vi "Dashboard Main.vi"() -> ()   [LabVIEW 2019]
uses:
  <vilib>/Utility/miscctls.llb/LVRowAndColumnTypeDef.ctl
  <vilib>/event_ctls.llb/eventvkey.ctl
  <vilib>/Rock Robotics/Network Tables/NT Read Numeric Array.vi
  <vilib>/Rock Robotics/WPI/Dashboard/WPI_DashboardLogging Global.vi
  <vilib>/Rock Robotics/Network Tables/NT Read Boolean.vi
panel:
  out "Conveyor Sensor 3":bool
  out "Conveyor Sensor 2":bool
  out "Conveyor Sensor 4":bool
  out "Conveyor Sensor 1":bool
  in  "Camera Settings Right":T1={"Frame Rate"=30, "Compression"=30, "Size"=1, "DB Camera Config"=FALSE} {"Frame Rate" scale=1.0..30.0; "Compression" scale=100.0..-1.0; "Size" items=["640x480", "320x240", "160x120"]}
  in  "Camera Name Right":string(combo)="No Camera Selection"
  out "Camera Perf":string
  in  "Camera Settings":T1={"Frame Rate"=30, "Compression"=30, "Size"=1, "DB Camera Config"=FALSE} {"Frame Rate" scale=1.0..30.0; "Compression" scale=100.0..-1.0; "Size" items=["640x480", "320x240", "160x120"]}
  in  "TCP":refnum<k5>
  in  "Rec Mode":enum32{"Stop", "Record", "Playback"}(radio)
  out "Robot IP":string
  out "Image Message":string="Timeout in Camera Communications"
  in  "Dashboard Tab":T2(tab)
  in  "Select Auto":string(combo)="Select Autonomous ..."
  out "NT Connection":bool
  out "MotorChart R":cluster{"Numeric":dbl, "Numeric":dbl}(graph)
  out "MotorChart L":cluster{"Numeric":dbl, "Numeric":dbl}(graph)
  out "MotorSliders R":cluster{"MotorSlide1":dbl, "MotorSlide2":dbl} {"MotorSlide2" scale=-1.0..1.0 scale format="%#_2e"; "MotorSlide1" scale=-1.0..1.0 scale format="%#_2e"}
  out "MotorSliders L":cluster{"MotorSlide1":dbl, "MotorSlide2":dbl} {"MotorSlide2" scale=-1.0..1.0 scale format="%#_2e"; "MotorSlide1" scale=-1.0..1.0 scale format="%#_2e"}
  out "JS1 Z":dbl(slide) scale=-1.0..1.0 scale format="%#_2e"
  out "JS1 Graph":cluster{"X":dbl, "Y":dbl}[](graph)
  out "JS1 Buttons":T3
  out "JS2 Z":dbl(slide) scale=-1.0..1.0 scale format="%#_2e"
  out "JS2 Graph":cluster{"X":dbl, "Y":dbl}[](graph)
  out "JS2 Buttons":T3
  out "Mode":T4(ring)=enum."Auto Disabled"
  out "Right Camera Perf":cluster{"Bandwidth (Mbps)":dbl, "FPS":dbl}
  out "Camera Image Right":T5(plugin-control)
  in  "DB/String 9":string
  in  "DB/String 8":string
  in  "DB/String 7":string
  in  "DB/String 6":string
  in  "DB/String 5":string
  in  "DB/String 4":string
  in  "DB/String 3":string
  in  "DB/String 2":string
  in  "DB/String 1":string
  in  "DB/String 0":string
  in  "DB/Slider 0":dbl(slide) scale=0.0..5.0
  in  "DB/Slider 1":dbl(slide) scale=0.0..5.0
  in  "DB/Slider 2":dbl(slide) scale=0.0..5.0
  in  "DB/Slider 3":dbl(slide) scale=0.0..5.0
  out "DB/LED 3":bool
  out "DB/LED 2":bool
  out "DB/LED 1":bool
  out "DB/LED 0":bool
  in  "DB/Button 3":bool
  in  "DB/Button 2":bool
  in  "DB/Button 1":bool
  in  "DB/Button 0":bool caption="New Name"
  in  "Right MP Path":path
  in  "Left MP Path":path
  in  "Test Slider":dbl(slide) scale=0.0..100.0 scale format="%#_3g"
  in  "On/Off":bool caption="Solenoid"
  in  "Test Name":u16(ring) items=["Select the test to run..."]
  in  "Test Tree":string(tree)
  in  "Motor":cluster{"Value":dbl, "Enable":bool} {"Value" scale=-1.0..1.0 scale format="%#_3g"}
  out "Progress":T6 {"Test Progress" scale=0.0..100.0}
  in  "Rev/Fwd":cluster{"Forward":bool, "Reverse":bool}
  in  "Test Ring":u16(ring) items=["Monochrome", "Color"]
  out "Cmd Status":string
  in  "Execute Command":bool
  in  "Command Params":string[][](table)
  in  "Command Selection":i32(listbox)
  in  "CheckList":i32(listbox)
  out "Tree":string(tree)
  out "Camera Image":T5(plugin-control)
  in  "Camera Name":string(combo)="No Camera Selection"
  # "HW"
  # "HW"
  # "Joysticks"
  # "Drive Motors"
  # "Front"
  # "Right"
  # "Left"
  # "Back"
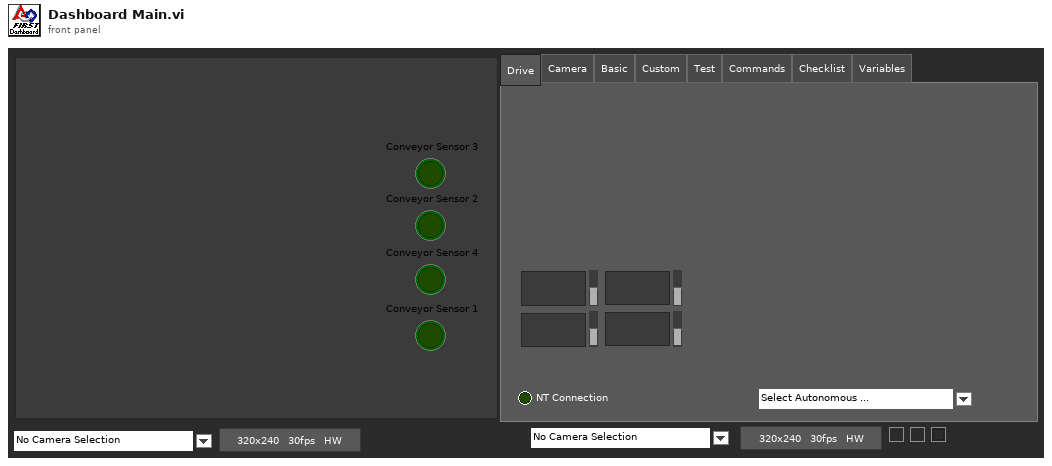
[diagram p1: front panel]
types:
  T1 = cluster{"Frame Rate":i32, "Compression":i32, "Size":u16, "DB Camera Config":bool}
  T2 = enum32{"Drive", "Camera", "Basic", "Custom", "Test", "Commands", "Checklist", "Variables"}
  T3 = cluster{bool, bool, bool, bool, bool, bool, bool, bool, bool, bool, bool, bool}
  T4 = enum8{"Tele-Op Disabled", "Tele-Op Enabled", "Auto Disabled", "Auto Enabled", "Test Disabled", "Test Enabled", "Disconnected", "No Code", "E-Stop"}
  T5 = typedef "IMAQ Image.ctl" = refnum<image>
  T6 = cluster{"Test Progress":u8, "Test Progress Text":string}
  T7 = enum16{"open", "replace", "create", "open or create", "replace or create", "replace or create with confirmation"}
  T8 = cluster{"Save Path":path, "Interval (s)":dbl, "Keep":i32}
  T9 = typedef "Image Type" = u32
  T10 = cluster{"IDs":cluster{"RPC field ID":u16, "Unique ID":u16}, "String":string}
  T11 = cluster{"Error Strings":string, "Disable Counts":cluster{u16, u16}, "Rail Faults":cluster{u16, u16, u16}, "Robot IP":string, "DB Mode":u8, "Event Info":cluster{"Name":string, "Type":u8, "Number":u16, "Replay":u8}}
  T12 = cluster{"Storage":cluster{"Disk Free":u64, "RAM Block":u32, "RAM free":u32}, "CPU Utilization":cluster{"CPU % ISR":sgl, "CPU % Time Crit":sgl, "CPU % Timed Str":sgl, "CPU % High":sgl, "CPU % Above":sgl, "CPU % Normal":sgl, "CPU % Low":sgl}, "CAN":cluster{"% Bus Utilization":sgl, "Bus Off Cnt":u32, "TX_FIFO Full Cnt":u32, "Receive Error Cnt":u8, "Transmit Error Cnt":u8}, "HID":cluster{"HID Outputs":u32, "Rumble Low":u16, "Rumble High":u16}[]}
  T13 = cluster{"Status bits":cluster{"Test Mode":bool, "Autonomous":bool, "Enabled":bool, "Code Start":bool, "Brownout":bool, "Reserved 2":bool, "Reserved 3":bool, "E-Stop":bool}, "Code Trace":cluster{"Disabled":bool, "TeleOp":bool, "Auto":bool, "Test":bool}, "Controller Type":enum16{"unknown", "cRIO", "roboRio"}, "Code?":enum16{"unknown", "noCode", "code"}, "Battery V":dbl}
  T14 = cluster{"Control Bits":cluster{"TestMode":bool, "Autonomous":bool, "Enabled":bool, "FMS Present":bool, bool, bool, bool, "E-Stop":bool}, "Team Station ":u8, "Countdown":sgl, "Joystick Values":cluster{"Axes":dbl[], "Buttons":bool[], "POVs":i16[]}[]}
  T15 = cluster{"Axes":dbl[], "Buttons":bool[], "POVs":i16[]}[]
  T16 = cluster{"Axes":dbl[], "Buttons":bool[], "POVs":i16[]}
  T17 = cluster{"Buttons[0]":bool, "Buttons[1]":bool, "Buttons[2]":bool, "Buttons[3]":bool, "Buttons[4]":bool, "Buttons[5]":bool, "Buttons[6]":bool, "Buttons[7]":bool, "Buttons[8]":bool, "Buttons[9]":bool, "Buttons[10]":bool, "Buttons[11]":bool}
  T18 = cluster{"Global Rectangle":i32[], "Contours":cluster{"Contour Type":u32, "ROI Type":u32, "Points":i32[]}[]}
  T19 = cluster{"Camera Name":string, string, "Saved DB Images Info":cluster{"Save Path":path, "Interval (s)":dbl, "Keep":i32}}
  T20 = cluster{"Camera Name Right":string, string, "Saved DB Images Info":cluster{"Save Path":path, "Interval (s)":dbl, "Keep":i32}}
  T21 = cluster{"Operation":enum16{"Update", "Clear"}, "Color Box":u32}[]
  T22 = typedef "eventvkey.ctl" = enum16{"ASCII", "Enter", "Return", "Shift", "Ctrl", "Alt", "Cmd", "Opt", "Caps", "NumLock", "Clear", "Break", "Up", "Down", "Left", "Right", "Insert", "Delete", "Home", "End", "PageUp", "PageDown", "Escape", "Help", "Pause", "ScrollLock", "F1", "F2", "F3", "F4", "F5", "F6", "F7", "F8", "F9", "F10", "F11", "F12", "F13", "F14", "F15", "F16", "F17", "F18", "F19", "F20", "F21", "F22", "F23", "F24", "Play", "VolumeUp", "VolumeDown", "Mute", "Two Byte Char"}
  T23 = cluster{"Image Size":bool, "Image Type":bool, "Pixel Value":bool, "ROI Information":bool, "Zoom Factor":bool}
  T24 = cluster{"Operation":enum16{"Update", "Clear"}, "Color Box":u32}
  T25 = typedef "LVRowAndColumnTypeDef.ctl" = cluster{"Row":i32, "Column":i32}
  T26 = cluster{"Shift":bool, "Ctrl":bool, "Alt":bool, "Cmd":bool, "Opt":bool}
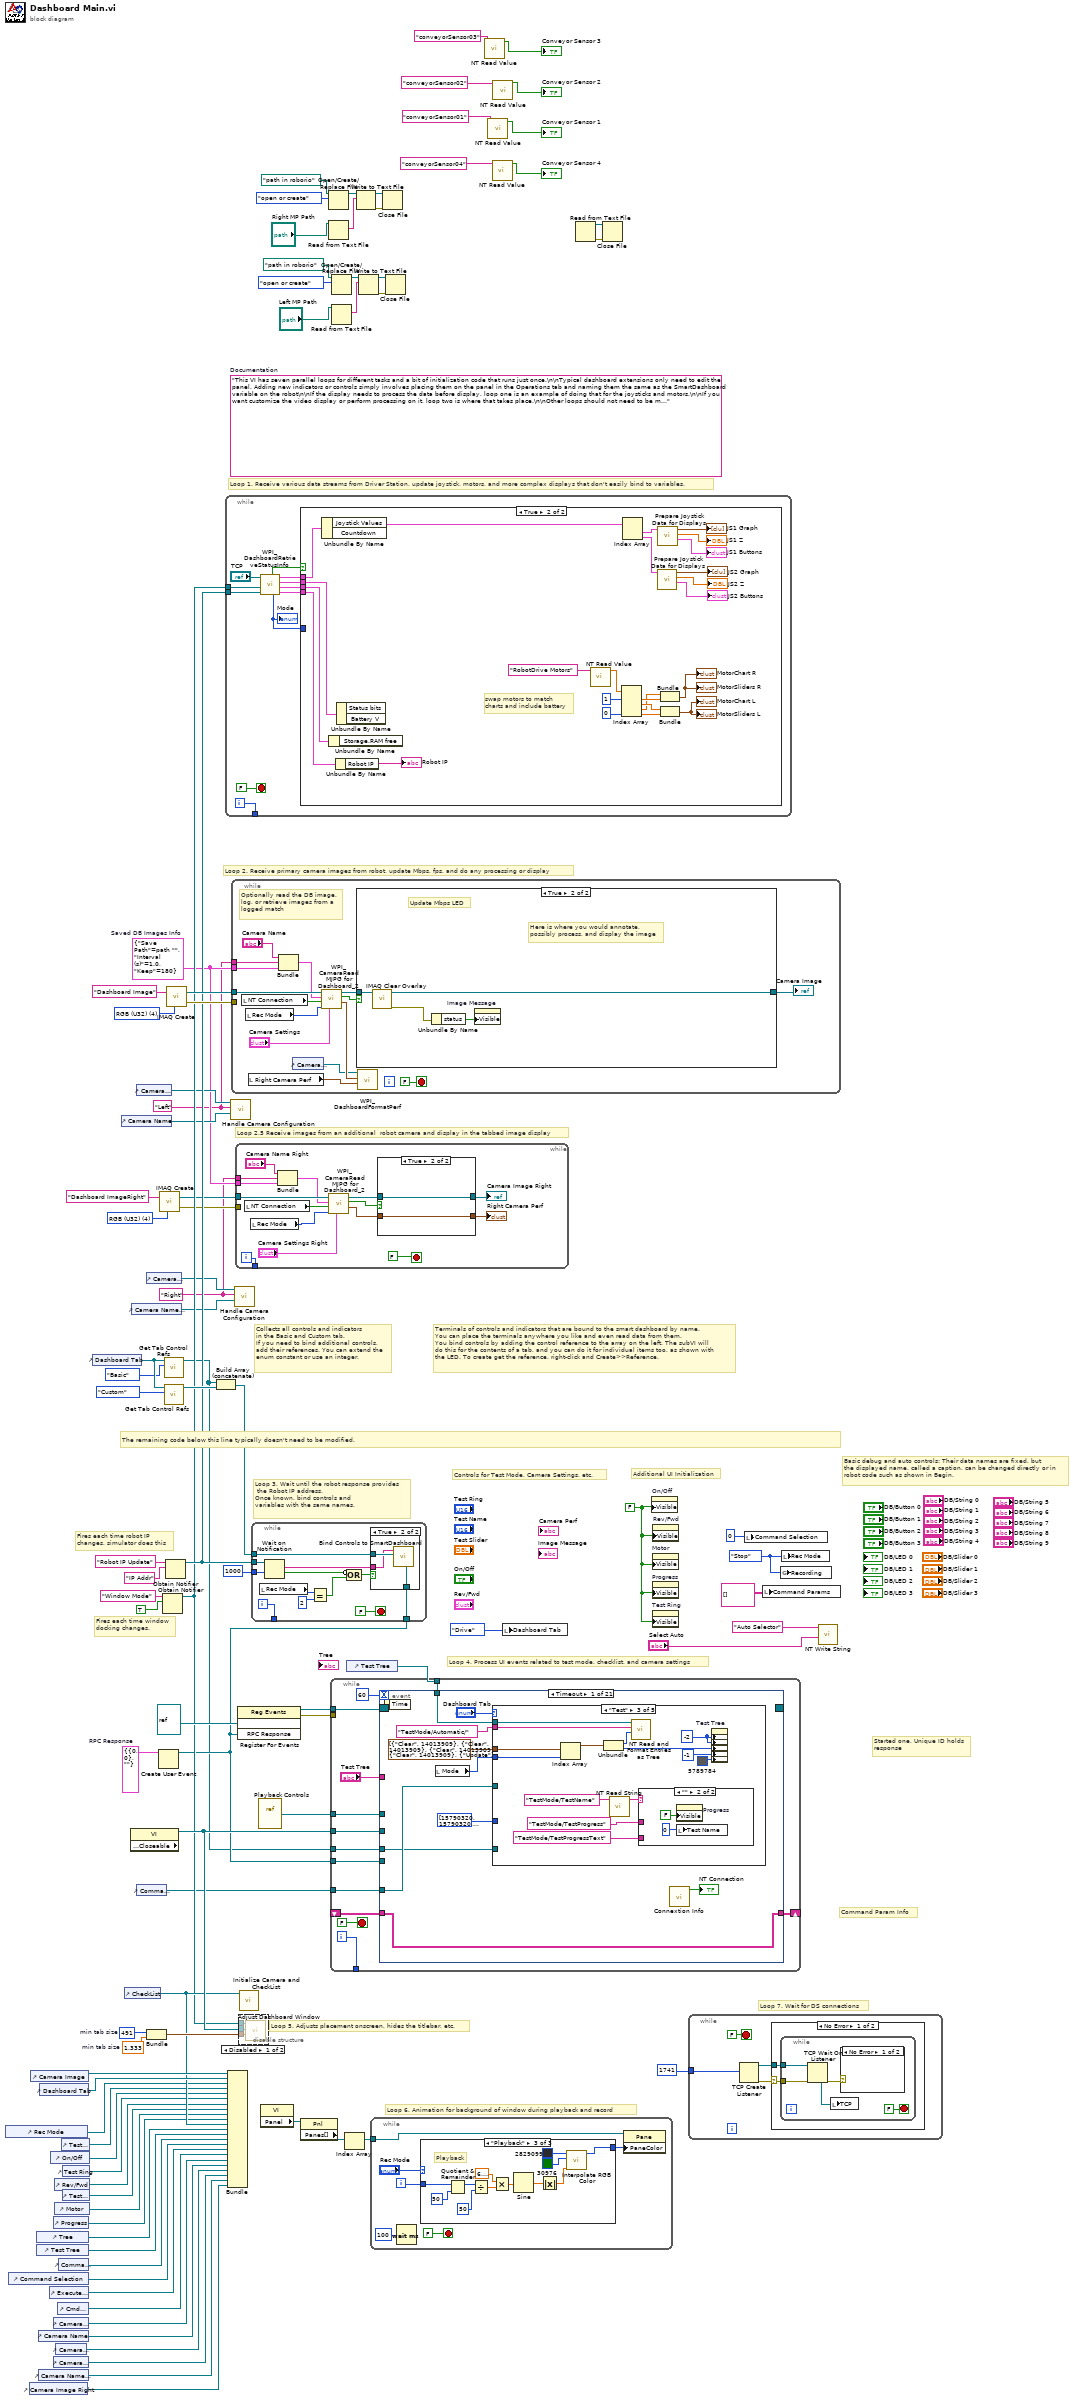
[diagram p0: block diagram]
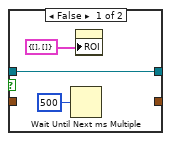
[diagram p3: hidden frame]
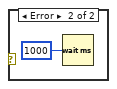
[diagram p4: hidden frame]
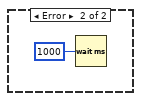
[diagram p5: hidden frame]
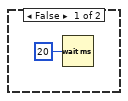
[diagram p6: hidden frame]
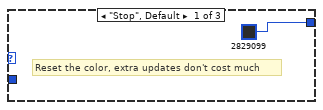
[diagram p7: hidden frame]
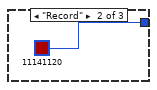
[diagram p8: hidden frame]
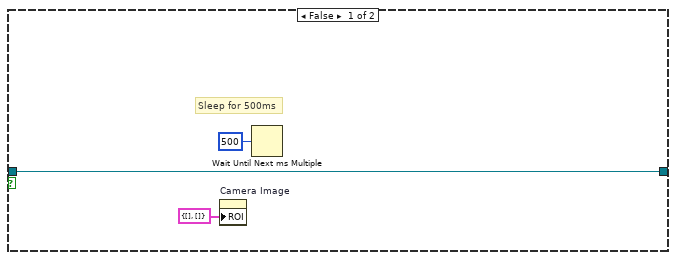
[diagram p10: hidden frame]
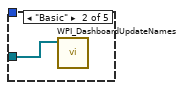
[diagram p12: hidden frame]
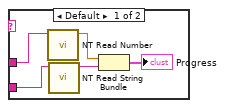
[diagram p13: hidden frame]
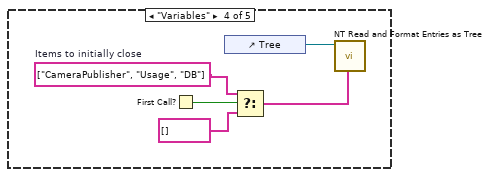
[diagram p14: hidden frame]
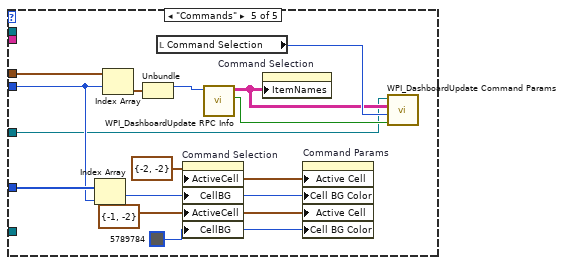
[diagram p15: hidden frame]
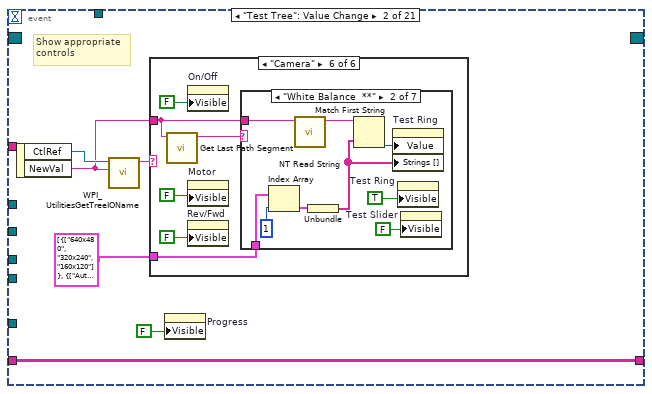
[diagram p16: hidden frame]
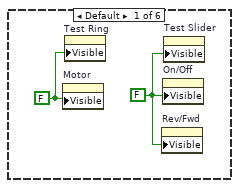
[diagram p17: hidden frame]
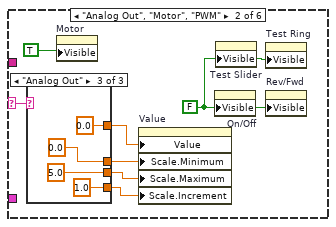
[diagram p18: hidden frame]
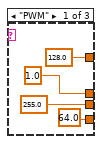
[diagram p19: hidden frame]
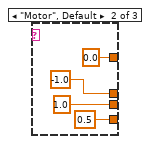
[diagram p20: hidden frame]
diagram:
  w27 = T8 {"Save Path"=path "", "Interval (s)"=1.0, "Keep"=180}  # Saved DB Images Info
  w26 = "Right"
  w25 = "Left"
  w37 = T9 4 items=["Grayscale (U8)", "Grayscale (I16)", "Grayscale (SGL)", "Complex (CSG)", "RGB (U32)", "HSL (U32)", "RGB (U64)"] ("Image Type")
  w53 = T10 {"IDs"={"RPC field ID"=0, "Unique ID"=0}, "String"=""}  # RPC Response
  w74 = 491  # min tab size
  w73 = 1.333  # min tab size
  w81 = enum32{"Stop", "Record", "Playback"}."Stop" ("Rec Mode")
  w60 = FALSE ("Visible")
  (unwired) "This VI has seven parallel loops for different tasks and a bit of initialization code that runs just once.\n\nTypical dashboard extensions only need to edit the panel. Adding new indicators or controls simply involves placing them on the panel in the Operations tab and naming them the same as the SmartDashboard variable on the robot\n\nIf the display needs to process the data before display, loop one is an example of doing that for the joysticks and motors.\n\nIf you want customize the video display or perform processing on it, loop two is where that takes place.\n\nOther loops should not need to be modified. They are pretty standard, and document the task they perform."  # Documentation
  w98 = T9 4 items=["Grayscale (U8)", "Grayscale (I16)", "Grayscale (SGL)", "Complex (CSG)", "RGB (U32)", "HSL (U32)", "RGB (U64)"] ("Image Type")
  # "Loop 2.5 Receive images from an additional  robot camera and display in the tabbed image display"
  # "Command Param Info"
  # "Started one, Unique ID holds\nresponse"
  # "Loop 7. Wait for DS connections"
  # "Basic debug and auto controls: Their data names are fixed, but\nthe displayed name, called a caption, can be changed directly or in\nrobot code such as shown in Begin."
  # "Controls for Test Mode, Camera Settings, etc."
  # "Additional UI Initialization"
  # "Loop 6. Animation for background of window during playback and record"
  # "Fires each time robot IP\nchanges, simulator does this"
  # "Fires each time window\ndocking changes."
  # "Collects all controls and indicators\nin the Basic and Custom tab.\nIf you need to bind additional controls,\nadd their references. You can extend the\nenum constant or use an integer."
  # "The remaining code below this line typically doesn't need to be modified."
  # "Loop 4. Process UI events related to test mode, checklist, and camera settings"
  # "Terminals of controls and indicators that are bound to the smart dashboard by name.\nYou can place the terminals anywhere you like and even read data from them.\nYou bind controls by adding the control reference to the array on the left. The subVI will\ndo this for the contents of a tab, and you can do it for individual items too, as shown with\nthe LED. To create get the reference, right-click and Create>>Reference."
  # "Loop 3. Wait until the robot response provides\n the Robot IP address.\nOnce known, bind controls and\nvariables with the same names."
  # "Loop 5. Adjusts placement onscreen, hides the titlebar, etc."
  # "Loop 1. Receive various data streams from Driver Station, update joystick, motors, and more complex displays that don't easily bind to variables."
  # "Loop 2. Receive primary camera images from robot, update Mbps, fps, and do any processing or display"
  n1 = control-ref of="Rec Mode"() -> (w66:refnum<vi>)
  n2 = control-ref of="Command Selection"() -> (w52:refnum<vi>)
  n3 = control-ref of="Camera Image Right"() -> (w30:refnum<vi>)
  n4 = control-ref of="Camera Image"() -> (w76:refnum<vi>)
  n5 = control-ref of="Tree"() -> (w70:refnum<vi>)
  n6 = control-ref of="Test Tree"() -> (w69:refnum<vi>)
  n7 = control-ref of="Camera Name"() -> (w43:refnum<vi>)
  n8 = control-ref of="Camera Name Right"() -> (w31:refnum<vi>)
  n9 = control-ref of="Dashboard Tab"() -> (w75:refnum<vi>)
  n10 = control-ref of="Execute Command"() -> (w54:refnum<vi>)
  n11 = control-ref of="On/Off"() -> (w64:refnum<vi>)
  n12 = control-ref of="Progress"() -> (w61:refnum<vi>)
  n13 = control-ref of="Camera Settings"() -> (w44:refnum<vi>)
  n14 = control-ref of="Camera Settings Right"() -> (w32:refnum<vi>)
  n15 = control-ref of="Rev/Fwd"() -> (w62:refnum<vi>)
  n16 = control-ref of="Motor"() -> (w67:refnum<vi>)
  n17 = control-ref of="Camera Perf"() -> (w42:refnum<vi>)
  n18 = control-ref of="Cmd Status"() -> (w48:refnum<vi>)
  n19 = control-ref of="Command Params"() -> (w55:refnum<vi>)
  n20 = control-ref of="Test Slider"() -> (w65:refnum<vi>)
  n21 = control-ref of="Test Ring"() -> (w63:refnum<vi>)
  n22 = control-ref of="Test Name"() -> (w68:refnum<vi>)
  n23 = control-ref of="Dashboard Tab"() -> (w79:refnum<vi>)
  n24 = control-ref of="Camera Name"() -> (w45:refnum<vi>)
  n25 = control-ref of="CheckList"() -> (w71:refnum<vi>)
  n26 = property class="VI" props=["Front Panel.Closeable"]() -> (reference out=w80:refnum<vi>)  [unwired: 2 in, 2 out]
  n27 = control-ref of="Camera Name Right"() -> (w33:refnum<vi>)
  n28 = control-ref of="Camera Settings"() -> (w46:refnum<vi>)
  n29 = control-ref of="Command Params"() -> (w47:refnum<vi>)
  n30 = control-ref of="Camera Settings Right"() -> (w34:refnum<vi>)
  n31 = Bundle("min tab size"=w74, "min tab size"=w73) -> (w72:cluster{"min tab size":i32, "min tab size":dbl})  [unwired: 1 in]
  n32 = Create User Event(user event datatype=w53) -> (user event=w49:refnum<user-event>)  [unwired: 1 in, 1 out]
  n33 = call "IMAQ Create"("Image Name"="Dashboard ImageRight", "Image Type"=w37) -> ("New Image"=w36:T5, "error out"=w35:errorcluster)  [unwired: 2 in, 1 out]
  n34 = Obtain Notifier(name (unnamed)="Window Mode", notification data type=TRUE) -> (notifier out=w58:refnum<notifier>)  [unwired: 2 in, 2 out]
  n35 = call <vilib>:"Get Tab Control Refs.vi"("Page Index"=T2."Basic" ("Dashboard Tab"), "TabControl in"=w79) -> ("ControlsOnPage"=w41:refnum<vi>[])  [unwired: 9 in]
  n36 = call <vilib>:"Get Tab Control Refs.vi"("Page Index"=T2."Custom" ("Dashboard Tab"), "TabControl in"=w79) -> ("ControlsOnPage"=w78:refnum<vi>[])  [unwired: 9 in]
  n37 = Obtain Notifier(name (unnamed)="Robot IP Update", notification data type="IP Addr" ("name (unnamed)")) -> (notifier out=w59:refnum<notifier>)  [unwired: 2 in, 2 out]
  n38 = call "IMAQ Create"("Image Name"="Dashboard Image", "Image Type"=w98) -> ("New Image"=w96:T5, "error out"=w95:errorcluster)  [unwired: 2 in, 1 out]
  n39 = Build Array (concatenate)(w41, w78) -> (w77:refnum<vi>[])
  n40 = while {
    tunnel: [w108] -> _
    tunnel: w59 -> [w102]
    tunnel: w58 -> [w99]
    i -> [w108]
    stop <- FALSE stop-if-true
    n41 = call <vilib>:"WPI_DashboardRetrieveStatusInfo.vi"("Binding Refnum"=w102, "Window Mode Notifier"=w99, "TCP Cnx"="TCP") -> ("Power and Errors"=w103:T11, "Robot Metrics"=w106:T12, "Status Info"=w107:T13, "Control Info"=w104:T14, "Robot Mode"=w101:T4, "Process?"=w105:bool)  [unwired: 3 in]
    "Mode" <- w101
    n42 = case shown="True" w105 {
      tunnel: w107 -> [_ w134]
      tunnel: w106 -> [_ w133]
      tunnel: w104 -> [_ w132]
      tunnel: w103 -> [_ w131]
      tunnel: w101 -> [_ _]
      frame False {
        n43 = Wait (ms)(milliseconds to wait=u32 20) -> ()  [unwired: 1 out]
      }
      frame True {
        # "swap motors to match\ncharts and include battery"
        n44 = Unbundle By Name(w132) -> ("Joystick Values"=w122:T15)  [unwired: 1 out]
        n45 = Unbundle By Name(w133) -> ()  [unwired: 1 out]
        n46 = Unbundle By Name(w131) -> ("Robot IP"=→"Robot IP":string)
        n47 = Unbundle By Name(w134) -> ()  [unwired: 2 out]
        n48 = call-poly <vilib>:"NT Read Value.vi"("Name"="RobotDrive Motors") -> ("Numeric Array"=w112:dbl[])  [unwired: 9 in, 1 out]
        n49 = Index Array(array=w112, index #1=1, index #4=0) -> (element #1=w126:dbl, element #2=w127:dbl, element #3=w125:dbl, element #4=w130:dbl)  [unwired: 2 in]
        n50 = Index Array(array=w122) -> (element #1=w121:T16, element #2=w117:T16)  [unwired: 2 in]
        n51 = call "Prepare Joystick Data for Displays.vi"("Joystick Values"=w117) -> ("Buttons"=→"JS2 Buttons":T17, "Z Axis"=→"JS2 Z":dbl, "Cartesian Data"=→"JS2 Graph":cluster{"X axis":dbl, "X axis":dbl}[])  [unwired: 8 in]
        n52 = call "Prepare Joystick Data for Displays.vi"("Joystick Values"=w121) -> ("Buttons"=→"JS1 Buttons":T17, "Z Axis"=→"JS1 Z":dbl, "Cartesian Data"=→"JS1 Graph":cluster{"X axis":dbl, "X axis":dbl}[])  [unwired: 8 in]
        n53 = Bundle("Numeric"=w125, "Numeric"=w126) -> (→"MotorChart R" →"MotorSliders R":cluster{"Numeric":dbl, "Numeric":dbl})  [unwired: 1 in]
        n54 = Bundle("Numeric"=w127, "Numeric"=w130) -> (→"MotorChart L" →"MotorSliders L":cluster{"Numeric":dbl, "Numeric":dbl})  [unwired: 1 in]
      }
    }
  }
  n55 = Bundle("Camera Image"=w76, "Dashboard Tab"=w75, "Rec Mode"=w66, "Test Slider"=w65, "On/Off"=w64, "Test Ring"=w63, "Rev/Fwd"=w62, "Test Name"=w68, "Motor"=w67, "Progress"=w61, "CheckList"=w71, "Tree"=w70, "Test Tree"=w69, "Command Params"=w55, "Command Selection"=w52, "Execute Command"=w54, "Cmd Status"=w48, "Camera Settings"=w44, "Camera Name"=w43, "Camera Perf"=w42, "Camera Settings Right"=w32, "Camera Name Right"=w31, "Camera Image Right"=w30) -> ()  [unwired: 1 in, 1 out]
  n56 = call "Handle Camera Configuration.vi"("CameraNameRef"=w45, "Display Name"=w25, "ClusterRef"=w46) -> ()  [unwired: 9 in]
  n57 = while {
    tunnel: w96 -> [w148]
    tunnel: w95 -> [_]
    tunnel: w27 -> [w141]
    tunnel: w25 -> [w138]
    stop <- FALSE stop-if-true
    # "Optionally read the DB image,\nlog, or retrieve images from a\nlogged match"
    n58 = local read "NT Connection"() -> (w142:bool)
    n59 = local read "Rec Mode"() -> (w145:enum32{"Stop", "Record", "Playback"})
    n60 = local read "Right Camera Perf"() -> (w136:cluster{"Bandwidth (Mbps)":dbl, "FPS":dbl})
    n61 = Bundle("Camera Name"="Camera Name", w138, "Saved DB Images Info"=w141) -> (w140:T19)  [unwired: 1 in]
    n62 = control-ref of="Camera Perf"() -> (w135:refnum<vi>)
    n63 = call <vilib>:"WPI_CameraRead MJPG for Dashboard_2.vi"("Camera Settings"="Camera Settings", "Rec Mode"=w145, "NT Connection"=w142, "Capture Info"=w140, "Image in"=w148) -> ("perf info"=w137:cluster{"Bandwidth (Mbps)":dbl, "fps":dbl}, "Active"=w146:bool, "Image\\ out"=w147:T5)  [unwired: 4 in]
    n64 = case shown="True" w146 {
      tunnel: w147 -> [w151 w154]
      tunnel: [w151 w153] -> w143
      frame False {
        # "Sleep for 500ms"
        n65 = property on="Camera Image" class="ImageControl"("ROI"=T18 {"Global Rectangle"=[], "Contours"=[]}) -> ()  [unwired: 2 in, 2 out]
        n66 = Wait Until Next ms Multiple(millisecond multiple=u32 500) -> ()  [unwired: 1 out]
      }
      frame True {
        # "Here is where you would annotate,\npossibly process, and display the image"
        # "Update Mbps LED"
        n67 = call "IMAQ Clear Overlay"("Image"=w154) -> ("error out"=w155:errorcluster, "Image Out"=w153:T5)  [unwired: 2 in, 7 out]
        n68 = Unbundle By Name(w155) -> ("status"=w156:bool)
        n69 = property on="Image Message" class="Str"("Visible"=w156) -> ()  [unwired: 2 in, 2 out]
      }
    }
    "Camera Image" <- w143
    n70 = call <vilib>:"WPI_DashboardFormatPerf.vi"("Right Camera Perf"=w136, "Performance"=w137, "String in"=w135) -> ()  [unwired: 9 in]
  }
  n71 = call "Handle Camera Configuration.vi"("CameraNameRef"=w33, "Display Name"=w26, "ClusterRef"=w34) -> ()  [unwired: 9 in]
  n72 = while {
    tunnel: w36 -> [w171]
    tunnel: w35 -> [_]
    tunnel: [w166] -> _
    tunnel: w27 -> [w162]
    tunnel: w26 -> [w159]
    i -> [w166]
    stop <- FALSE stop-if-true
    n73 = local read "NT Connection"() -> (w163:bool)
    n74 = local read "Rec Mode"() -> (w170:enum32{"Stop", "Record", "Playback"})
    n75 = Bundle("Camera Name Right"="Camera Name Right", w159, "Saved DB Images Info"=w162) -> (w161:T20)  [unwired: 1 in]
    n76 = call <vilib>:"WPI_CameraRead MJPG for Dashboard_2.vi"("Camera Settings"="Camera Settings Right", "Rec Mode"=w170, "NT Connection"=w163, "Capture Info"=w161, "Image in"=w171) -> ("perf info"=w157:cluster{"Bandwidth (Mbps)":dbl, "fps":dbl}, "Active"=w165:bool, "Image\\ out"=w168:T5)  [unwired: 4 in]
    n77 = case shown="True" w165 {
      tunnel: w168 -> [w173 w176]
      tunnel: [w173 w176] -> w164
      tunnel: [_ w175] -> w158
      tunnel: w157 -> [_ w175]
      frame False {
        n78 = Wait Until Next ms Multiple(millisecond multiple=u32 500) -> ()  [unwired: 1 out]
        n79 = property on="Camera Image Right" class="ImageControl"("ROI"=T18 {"Global Rectangle"=[], "Contours"=[]}) -> ()  [unwired: 2 in, 2 out]
      }
      frame True {
      }
    }
    "Camera Image Right" <- w164
    "Right Camera Perf" <- w158
  }
  n80 = register-events(refnum<vi> refnum, w49) -> (reference out=w85:refnum<event-registration>, error out=w84:errorcluster)  [unwired: 2 in]
  n81 = disable-structure shown="Disabled" {
    disable-tunnel: w80 -> [w179 _]
    disable-tunnel: w72 -> [w178 _]
    disable-tunnel: w58 -> [w177 _]
    frame Disabled {
      n82 = call "Adjust Dashboard Window.vi"("Size Constraints"=w178, "VI"=w179, "WIn Mode"=w177) -> ()  [unwired: 9 in]
    }
    frame Enabled {
    }
  }
  n83 = call "Initialize Camera and CheckList.vi"("ListBox in"=w71) -> ()  [unwired: 11 in]
  n84 = while {
    tunnel: w77 -> [w191]
    tunnel: w59 -> [w189]
    tunnel: [w187] -> _
    tunnel: u32 1000 ("milliseconds to wait") -> [w186]
    tunnel: w49 -> [w180]
    i -> [w187]
    stop <- FALSE stop-if-true
    n85 = local read "Rec Mode"() -> (w182:enum32{"Stop", "Record", "Playback"})
    n86 = Wait on Notification(notifier=w189, timeout in ms (-1)=w186) -> (notification=w188:string, timed out?=w184:bool)  [unwired: 2 in, 2 out]
    n87 = Equal?(x=w182, y=u16 2 ("Rec Mode")) -> (x = y?=w183:bool)
    n88 = Compound Arithmetic op=OR(invert w184, w183) -> (w185:bool)
    n89 = case shown="True" w185 {
      tunnel: w191 -> [_ w194]
      tunnel: w188 -> [_ w193]
      tunnel: w180 -> [_ w192]
      frame False {
      }
      frame True {
        n90 = call <vilib>:"Bind Controls to SmartDashboard.vi"("RPC ref"=w192, "Bound Control Refs"=w194, "Server IP Address"=w193) -> ()  [unwired: 9 in]
      }
    }
  }
  n91 = vi-ref "Playback Controls.vi"() -> (w86:refnum<vi>)
  n92 = property class="VI"() -> ("Panel"=w88:refnum<vi>)  [unwired: 2 in, 2 out]
  n93 = property class="Pnl"(reference=w88) -> ("Panes[]"=w89:refnum<vi>[])  [unwired: 1 in, 2 out]
  n94 = Open/Create/Replace File(file path (use dialog)=path "path in roborio", operation (0:open)=T7."open or create") -> (refnum out=w23:refnum<file>)  [unwired: 4 in, 2 out]
  n95 = Read from Text File(file (use dialog)="Right MP Path") -> (text=w20:string)  [unwired: 3 in, 3 out]
  n96 = Open/Create/Replace File(file path (use dialog)=path "path in roborio", operation (0:open)=T7."open or create") -> (refnum out=w17:refnum<file>)  [unwired: 4 in, 2 out]
  n97 = Read from Text File(file (use dialog)="Left MP Path") -> (text=w15:string)  [unwired: 3 in, 3 out]
  n98 = Index Array(array=w89) -> (element=w87:refnum<vi>)  [unwired: 1 in]
  n99 = control-ref of="Test Tree"() -> (w90:refnum<vi>)
  n100 = while {
    tunnel: [w204] -> _
    tunnel: w90 -> [w203]
    tunnel: w86 -> [w202]
    tunnel: w85 -> [w201]
    tunnel: w84 -> [_]
    tunnel: w80 -> [w200]
    tunnel: w49 -> [w199]
    tunnel: w47 -> [w198]
    shift-right: [w197] -> _
    shift-left: _ -> [w196]
    tunnel: w41 -> [w195]
    i -> [w204]
    stop <- FALSE stop-if-true
    n101 = event shown="[0] Timeout" {
      selector: w201 -> [_ _ _ _ _ _ _ _ _ _ _ _ _ _ _ _ _ _ _ _ _]
      dyn-events: [_ _ _ _ _ _ _ _ _ _ _ _ _ _ _ _ w464 _ _ _ _] -> _
      timeout: u32 60 ("milliseconds to wait") -> [_ _ _ _ _ _ _ _ _ _ _ _ _ _ _ _ _ _ _ _ _]
      tunnel: w203 -> [w216 _ _ _ _ _ _ _ _ _ _ _ _ _ _ _ _ _ _ _ _]
      tunnel: "Test Tree" -> [_ _ _ _ _ _ _ _ _ _ _ w431 w439 w441 w445 w453 _ _ _ _ _]
      tunnel: w202 -> [_ _ _ _ _ _ _ _ _ _ _ _ _ _ _ _ w466 _ w484 _ _]
      tunnel: w200 -> [_ _ _ _ _ _ _ _ _ _ _ _ _ _ _ _ w462 _ _ _ _]
      tunnel: w199 -> [_ _ _ _ _ _ _ _ _ _ _ _ _ _ _ _ w460 _ _ _ _]
      tunnel: w198 -> [w211 _ _ _ _ _ w382 _ _ _ _ _ _ _ _ _ _ _ _ _ _]
      tunnel: [w210 w259 w361 w366 w375 w379 w380 w389 w399 w406 w418 w430 w437 w440 w444 w452 w459 w479 w481 w485 w498] -> w197
      tunnel: w196 -> [w210 w259 w361 w366 w375 w379 w380 _ _ w406 w418 w430 w437 w440 w444 w452 w459 w479 w481 w485 w498]
      tunnel: w195 -> [w208 _ _ _ _ _ _ _ _ _ _ _ _ _ _ _ _ _ _ _ _]
      event Timeout {
        n102 = event-data() -> ()  [unwired: 1 in, 1 out]
        n103 = local read "Mode"() -> (w213:T4)
        n104 = case shown="\"Test\"" "Dashboard Tab" {
          tunnel: w216 -> [_ _ w232 _ _]
          tunnel: "TestMode/Automatic/" ("Name Pattern") -> [_ _ w231 _ _]
          tunnel: T21 [{"Operation"=enum."Clear", "Color Box"=14013909}, {"Operation"=enum."Clear", "Color Box"=14013909}, {"Operation"=enum."Clear", "Color Box"=14013909}, {"Operation"=enum."Clear", "Color Box"=14013909}, {"Operation"=enum."Update", "Color Box"=14013909}, {"Operation"=enum."Update", "Color Box"=16777215}, {"Operation"=enum."Clear", "Color Box"=14013909}, {"Operation"=enum."Clear", "Color Box"=14013909}, {"Operation"=enum."Clear", "Color Box"=14013909}] -> [_ _ w224 _ w252]
          tunnel: w213 -> [_ _ w223 _ w251]
          tunnel: u32[] [15790320, 15790320, 15790320, 15790320, 16777215, 16777215, 15790320, 15790320, 15790320] -> [_ _ _ _ w257]
          tunnel: w211 -> [_ _ _ _ w245]
          tunnel: w208 -> [_ w218 _ _ _]
          frame "Custom", Default {
          }
          frame "Basic" {
            n105 = call <vilib>:"WPI_DashboardUpdateNames.vi"("Controls on Tab"=w218) -> ()  [unwired: 11 in]
          }
          frame "Test" {
            w230 = -2 ("Active Item:Row Number")
            n106 = Index Array(array=w224, index=w223) -> (element=w225:T24)
            n107 = Unbundle(w225) -> ("Operation"=w226:enum16{"Update", "Clear"}, "Color Box"=w227:u32)
            n108 = call <vilib>:"NT Read String.vi"("Name"="TestMode/TestName") -> ("String"=w221:string)  [unwired: 9 in, 1 out]
            n109 = call <vilib>:"NT Read and Format Entries as Tree.vi"("Operation"=w226, "Name Pattern"=w231, "Tree Refnum"=w232) -> ()  [unwired: 7 in, 2 out]
            n110 = case shown="\"\"" w221 {
              tunnel: "TestMode/TestProgress" ("Name") -> [w234 _]
              tunnel: "TestMode/TestProgressText" ("Name") -> [w233 _]
              frame Default {
                n111 = call <vilib>:"NT Read Number.vi"("Name"=w234) -> ("Numeric"=w235:dbl)  [unwired: 9 in, 1 out]
                n112 = call <vilib>:"NT Read String.vi"("Name"=w233) -> ("String"=w236:string)  [unwired: 9 in, 1 out]
                n113 = Bundle("Numeric"=w235, "String"=w236) -> (→"Progress":cluster{"Numeric":dbl, "String":string})  [unwired: 1 in]
              }
              frame "" {
                n114 = property on="Progress" class="Clust (strict)"("Visible"=FALSE) -> ()  [unwired: 2 in, 2 out]
                n115 = local write "Test Name"(u16 0) -> ()
              }
            }
            n116 = property on="Test Tree" class="Tree (strict)"("Active Item Row Number"=w230, "ActiveColNum"=w230, "CellBG"=w227, "Active Item Row Number"=-1 ("Active Item:Row Number"), "CellBG"=u32 5789784 ("Color Box")) -> ()  [unwired: 2 in, 2 out]
          }
          frame "Variables" {
            w242 = string[] ["CameraPublisher", "Usage", "DB"]  # Items to initially close
            n117 = First Call?() -> (First Call?: T/F=w243:bool)
            n118 = control-ref of="Tree"() -> (w244:refnum<vi>)
            n119 = Select(t=w242, s=w243, f=string[] []) -> (s? t:f=w240:string[])
            n120 = call <vilib>:"NT Read and Format Entries as Tree.vi"("Tags to  Close"=w240, "Tree Refnum"=w244) -> ()  [unwired: 8 in, 2 out]
          }
          frame "Commands" {
            w253 = u32 5789784 ("Color Box")
            w254 = T25 {"Row"=-1, "Column"=-2} ("Active Cell:Active Cell")
            w256 = T25 {"Row"=-2, "Column"=-2} ("Active Cell:Active Cell")
            n121 = Index Array(array=w257, index=w251) -> (element=w255:u32)
            n122 = Index Array(array=w252, index=w251) -> (element=w250:T24)
            n123 = Unbundle(w250) -> ("Operation"=w249:enum16{"Update", "Clear"})  [unwired: 1 out]
            n124 = local read "Command Selection"() -> (w248:i32)
            n125 = property on="Command Selection" class="MCListbox (strict)"("ActiveCell"=w256, "CellBG"=w255, "ActiveCell"=w254, "CellBG"=w253) -> ()  [unwired: 2 in, 2 out]
            n126 = call <vilib>:"WPI_DashboardUpdate RPC Info.vi"("Operation"=w249) -> ("update"=w247:bool, "commands"=w246:string[][])  [unwired: 9 in]
            n127 = property on="Command Selection" class="MCListbox (strict)"("ItemNames"=w246) -> ()  [unwired: 2 in, 2 out]
            n128 = property on="Command Params" class="Tbl (strict)"("Active Cell"=w256, "Cell BG Color"=w255, "Active Cell"=w254, "Cell BG Color"=w253) -> ()  [unwired: 2 in, 2 out]
            n129 = call <vilib>:"WPI_DashboardUpdate Command Params.vi"("Update"=w247, "NewVal"=w248, "Commands"=w246, "Param Tbl"=w245) -> ()  [unwired: 7 in, 1 out]
          }
        }
        n130 = call <vilib>:"Connextion Info.vi"() -> ("Connected"=→"NT Connection":bool)  [unwired: 10 in, 1 out]
      }
      event "Test Tree": Value Change {
        # "Show appropriate\ncontrols"
        n131 = event-data() -> ("CtlRef"=w262:refnum<vi>, "NewVal"=w260:string)  [unwired: 1 in]
        n132 = call <vilib>:"WPI_UtilitiesGetTreeIOName.vi"("NewVal"=w260, "TreeControl in"=w262) -> ("I/O Name"=w263:string)  [unwired: 9 in]
        n133 = case shown="\"Camera\"" w263 {
          selector: w263 -> [_ w270 _ w292 w301 _]
          tunnel: w260 -> [_ _ w289 w291 _ w308]
          tunnel: cluster{string[]}[] [{["640x480", "320x240", "160x120"]}, {["Auto", "Fixed indoor", "Fixed outdoor 1", "Fixed outdoor 2", "Fixed fluorescent 1", "Fixed fluorescent 2", "Hold current"]}, {["Auto", "Flicker-free 50 Hz", "Flicker-free 60 Hz", "Hold current"]}, {["None", "Prioritize frame rate", "Prioritize image quality"]}, {["Monochrome", "Color"]}] -> [_ _ _ _ _ w307]
          frame Default {
            w265 = FALSE ("Visible")
            w264 = FALSE ("Visible")
            n134 = property on="Motor" class="Clust (strict)"("Visible"=w264) -> ()  [unwired: 2 in, 2 out]
            n135 = property on="Test Ring" class="Ring (strict)"("Visible"=w264) -> ()  [unwired: 2 in, 2 out]
            n136 = property on="Rev/Fwd" class="Clust (strict)"("Visible"=w265) -> ()  [unwired: 2 in, 2 out]
            n137 = property on="On/Off" class="Bool (strict)"("Visible"=w265) -> ()  [unwired: 2 in, 2 out]
            n138 = property on="Test Slider" class="Slide (strict)"("Visible"=w265) -> ()  [unwired: 2 in, 2 out]
          }
          frame "Analog Out", "Motor", "PWM" {
            w271 = FALSE ("Visible")
            n139 = case shown="\"Analog Out\"" w270 {
              tunnel: [1.0 ("Value") -1.0 ("Value") 0.0 ("Value")] -> w269
              tunnel: [255.0 ("Value") 1.0 ("Value") 5.0 ("Value")] -> w268
              tunnel: [128.0 ("Value") 0.0 ("Value") 0.0 ("Value")] -> w267
              tunnel: [64.0 ("Value") 0.5 ("Value") 1.0 ("Value")] -> w266
              frame "PWM" {
              }
              frame "Motor", Default {
              }
              frame "Analog Out" {
              }
            }
            n140 = property on="Motor" class="Clust (strict)"("Visible"=TRUE) -> ()  [unwired: 2 in, 2 out]
            n141 = property on="Value" class="Slide (strict)"("Value"=w267, "Scale.Minimum"=w269, "Scale.Maximum"=w268, "Scale.Increment"=w266) -> ()  [unwired: 2 in, 2 out]
            n142 = property on="On/Off" class="Bool (strict)"("Visible"=w271) -> ()  [unwired: 2 in, 2 out]
            n143 = property on="Test Slider" class="Slide (strict)"("Visible"=w271) -> ()  [unwired: 2 in, 2 out]
            n144 = property on="Test Ring" class="Ring (strict)"("Visible"=w271) -> ()  [unwired: 2 in, 2 out]
            n145 = property on="Rev/Fwd" class="Clust (strict)"("Visible"=w271) -> ()  [unwired: 2 in, 2 out]
          }
          frame "Servo" {
            w287 = FALSE ("Visible")
            n146 = call <vilib>:"NT Read Number.vi"("Name"=w289) -> ("Numeric"=w288:dbl)  [unwired: 9 in, 1 out]
            n147 = property on="Test Slider" class="Slide (strict)"("Visible"=TRUE, "Scale.Maximum"=170.0 ("Scale.Range:Maximum")) -> ()  [unwired: 2 in, 2 out]
            n148 = local write "Test Slider"(w288) -> ()
            n149 = property on="Motor" class="Clust (strict)"("Visible"=w287) -> ()  [unwired: 2 in, 2 out]
            n150 = property on="Rev/Fwd" class="Clust (strict)"("Visible"=w287) -> ()  [unwired: 2 in, 2 out]
            n151 = property on="On/Off" class="Bool (strict)"("Visible"=w287) -> ()  [unwired: 2 in, 2 out]
            n152 = property on="Test Ring" class="Ring (strict)"("Visible"=w287) -> ()  [unwired: 2 in, 2 out]
          }
          frame "Relay", "Solenoid" {
            w290 = FALSE ("Visible")
            n153 = property on="Motor" class="Clust (strict)"("Visible"=w290) -> ()  [unwired: 2 in, 2 out]
            n154 = property on="Test Slider" class="Slide (strict)"("Visible"=w290) -> ()  [unwired: 2 in, 2 out]
            n155 = Search and Replace String(input string=w291, search string="/Value  **", replace string="/Direction") -> (result string=w297:string)  [unwired: 5 in, 3 out]
            n156 = property on="Test Ring" class="Ring (strict)"("Visible"=w290) -> ()  [unwired: 2 in, 2 out]
            n157 = call <vilib>:"NT Read String.vi"("Name"=w297) -> ("String"=w295:string)  [unwired: 9 in, 1 out]
            n158 = Equal?(x="Both directions", y=w295) -> (x = y?=w293:bool)
            n159 = Not(x=w293) -> (.not. x?=w294:bool)
            n160 = property on="Rev/Fwd" class="Clust (strict)"("Visible"=w293) -> ()  [unwired: 2 in, 2 out]
            n161 = property on="On/Off" class="Bool (strict)"("Visible"=w294, "Caption.Text"=w292) -> ()  [unwired: 2 in, 2 out]
          }
          frame "Compressor", "Digital Out" {
            w300 = FALSE ("Visible")
            # "Get direction and finish"
            n162 = property on="Motor" class="Clust (strict)"("Visible"=w300) -> ()  [unwired: 2 in, 2 out]
            n163 = property on="Test Slider" class="Slide (strict)"("Visible"=w300) -> ()  [unwired: 2 in, 2 out]
            n164 = property on="Test Ring" class="Ring (strict)"("Visible"=w300) -> ()  [unwired: 2 in, 2 out]
            n165 = property on="On/Off" class="Bool (strict)"("Visible"=TRUE, "Caption.Text"=w301) -> ()  [unwired: 2 in, 2 out]
            n166 = property on="Rev/Fwd" class="Clust (strict)"("Visible"=FALSE) -> ()  [unwired: 2 in, 2 out]
          }
          frame "Camera" {
            n167 = call <vilib>:"Get Last Path Segment.vi"("String in"=w308) -> ("String out"=w309:string)  [unwired: 10 in]
            n168 = property on="On/Off" class="Bool (strict)"("Visible"=FALSE) -> ()  [unwired: 2 in, 2 out]
            n169 = property on="Motor" class="Clust (strict)"("Visible"=FALSE) -> ()  [unwired: 2 in, 2 out]
            n170 = property on="Rev/Fwd" class="Clust (strict)"("Visible"=FALSE) -> ()  [unwired: 2 in, 2 out]
            n171 = case shown="\"White Balance  **\"" w309 {
              tunnel: w308 -> [w315 w324 w333 w342 w351 _ w357]
              tunnel: w307 -> [w313 w321 w330 w339 w348 _ _]
              frame "Size  **" {
                n172 = Index Array(array=w313) -> (element=w312:cluster{string[]})  [unwired: 1 in]
                n173 = call <vilib>:"NT Read String.vi"("Name"=w315) -> ("String"=w314:string)  [unwired: 9 in, 1 out]
                n174 = Unbundle(w312) -> (w310:string[])
                n175 = Match First String(2:w310, 3:w314) -> (0:w311:i32)  [unwired: 1 out]
                n176 = property on="Test Ring" class="Ring (strict)"("Value"=w311, "Strings []"=w310) -> ()  [unwired: 2 in, 2 out]
                n177 = property on="Test Ring" class="Ring (strict)"("Visible"=TRUE) -> ()  [unwired: 2 in, 2 out]
                n178 = property on="Test Slider" class="Slide (strict)"("Visible"=FALSE) -> ()  [unwired: 2 in, 2 out]
              }
              frame "White Balance  **" {
                n179 = Index Array(array=w321, index=1) -> (element=w322:cluster{string[]})
                n180 = call <vilib>:"NT Read String.vi"("Name"=w324) -> ("String"=w323:string)  [unwired: 9 in, 1 out]
                n181 = Unbundle(w322) -> (w319:string[])
                n182 = Match First String(2:w319, 3:w323) -> (0:w318:i32)  [unwired: 1 out]
                n183 = property on="Test Ring" class="Ring (strict)"("Value"=w318, "Strings []"=w319) -> ()  [unwired: 2 in, 2 out]
                n184 = property on="Test Ring" class="Ring (strict)"("Visible"=TRUE) -> ()  [unwired: 2 in, 2 out]
                n185 = property on="Test Slider" class="Slide (strict)"("Visible"=FALSE) -> ()  [unwired: 2 in, 2 out]
              }
              frame "Exposure  **" {
                n186 = Index Array(array=w330, index=2) -> (element=w331:cluster{string[]})
                n187 = call <vilib>:"NT Read String.vi"("Name"=w333) -> ("String"=w332:string)  [unwired: 9 in, 1 out]
                n188 = Unbundle(w331) -> (w327:string[])
                n189 = Match First String(2:w327, 3:w332) -> (0:w328:i32)  [unwired: 1 out]
                n190 = property on="Test Ring" class="Ring (strict)"("Value"=w328, "Strings []"=w327) -> ()  [unwired: 2 in, 2 out]
                n191 = property on="Test Ring" class="Ring (strict)"("Visible"=TRUE) -> ()  [unwired: 2 in, 2 out]
                n192 = property on="Test Slider" class="Slide (strict)"("Visible"=FALSE) -> ()  [unwired: 2 in, 2 out]
              }
              frame "Exposure Priority  **" {
                n193 = Index Array(array=w339, index=3) -> (element=w340:cluster{string[]})
                n194 = call <vilib>:"NT Read String.vi"("Name"=w342) -> ("String"=w341:string)  [unwired: 9 in, 1 out]
                n195 = Unbundle(w340) -> (w336:string[])
                n196 = Match First String(2:w336, 3:w341) -> (0:w337:i32)  [unwired: 1 out]
                n197 = property on="Test Ring" class="Ring (strict)"("Value"=w337, "Strings []"=w336) -> ()  [unwired: 2 in, 2 out]
                n198 = property on="Test Ring" class="Ring (strict)"("Visible"=TRUE) -> ()  [unwired: 2 in, 2 out]
                n199 = property on="Test Slider" class="Slide (strict)"("Visible"=FALSE) -> ()  [unwired: 2 in, 2 out]
              }
              frame "Color Enable  **" {
                n200 = Index Array(array=w348, index=4) -> (element=w349:cluster{string[]})
                n201 = call <vilib>:"NT Read String.vi"("Name"=w351) -> ("String"=w350:string)  [unwired: 9 in, 1 out]
                n202 = Unbundle(w349) -> (w345:string[])
                n203 = Match First String(2:w345, 3:w350) -> (0:w346:i32)  [unwired: 1 out]
                n204 = property on="Test Ring" class="Ring (strict)"("Value"=w346, "Strings []"=w345) -> ()  [unwired: 2 in, 2 out]
                n205 = property on="Test Ring" class="Ring (strict)"("Visible"=TRUE) -> ()  [unwired: 2 in, 2 out]
                n206 = property on="Test Slider" class="Slide (strict)"("Visible"=FALSE) -> ()  [unwired: 2 in, 2 out]
              }
              frame Default {
                n207 = property on="Test Ring" class="Ring (strict)"("Visible"=FALSE) -> ()  [unwired: 2 in, 2 out]
                n208 = property on="Test Slider" class="Slide (strict)"("Visible"=FALSE) -> ()  [unwired: 2 in, 2 out]
              }
              frame "Brightness  **", "Color Level  **", "Compression  **", "FPS  **", "Sharpness  **" {
                n209 = call <vilib>:"NT Read Number.vi"("Name"=w357) -> ("Numeric"=w356:dbl)  [unwired: 9 in, 1 out]
                n210 = local write "Test Slider"(w356) -> ()
                n211 = property on="Test Slider" class="Slide (strict)"("Visible"=TRUE, "Scale.Maximum"=100.0 ("Scale.Range:Maximum")) -> ()  [unwired: 2 in, 2 out]
                n212 = property on="Test Ring" class="Ring (strict)"("Visible"=FALSE) -> ()  [unwired: 2 in, 2 out]
              }
            }
          }
        }
        n213 = property on="Progress" class="Clust (strict)"("Visible"=FALSE) -> ()  [unwired: 2 in, 2 out]
      }
      event "Test Name": Mouse Enter {
        # "Populate the ring with the list of tests"
        n214 = event-data() -> ()  [unwired: 1 in, 1 out]
        n215 = call <vilib>:"NT Read String Array.vi"("Name"="TestMode/TestList") -> ("String Array"=w365:string[])  [unwired: 9 in, 1 out]
        n216 = Build Array (concatenate)("Select the test to run...", w365) -> (w364:string[])
        n217 = property on="Test Name" class="Ring (strict)"("Strings []"=w364) -> ()  [unwired: 2 in, 2 out]
      }
      event "Test Name": Value Change {
        w367 = FALSE ("Visible")
        # "Tell the robot the test name to run"
        n218 = event-data() -> ("NewVal"=w371:u16)  [unwired: 1 in]
        n219 = property on="Test Name" class="Ring (strict)"() -> ("Strings []"=w372:string[])  [unwired: 2 in, 2 out]
        n220 = local write "Progress"(T6 {"Test Progress"=0, "Test Progress Text"=""} ("Progress")) -> ()
        n221 = Index Array(array=w372, index=w371) -> (element=w370:string)
        n222 = call <vilib>:"NT Write String.vi"("String"=w370, "Name"="TestMode/TestName") -> ()  [unwired: 9 in, 1 out]
        n223 = property on="Progress" class="Clust (strict)"("Visible"=TRUE) -> ()  [unwired: 2 in, 2 out]
        n224 = property on="Motor" class="Clust (strict)"("Visible"=w367) -> ()  [unwired: 2 in, 2 out]
        n225 = property on="Test Slider" class="Slide (strict)"("Visible"=w367) -> ()  [unwired: 2 in, 2 out]
        n226 = property on="On/Off" class="Bool (strict)"("Visible"=w367) -> ()  [unwired: 2 in, 2 out]
        n227 = property on="Rev/Fwd" class="Clust (strict)"("Visible"=w367) -> ()  [unwired: 2 in, 2 out]
        n228 = property on="Test Ring" class="Ring (strict)"("Visible"=w367) -> ()  [unwired: 2 in, 2 out]
      }
      event "Select Auto": Mouse Enter {
        # "Populate the combo box with the list of autonomous options"
        n229 = event-data() -> ()  [unwired: 1 in, 1 out]
        n230 = call <vilib>:"NT Read String Array.vi"("Name"="Auto List") -> ("String Array"=w374:string[])  [unwired: 9 in, 1 out]
        n231 = property on="Select Auto" class="CmbBox"("Strings[]"=w374) -> ()  [unwired: 2 in, 2 out]
      }
      event "Select Auto": Value Change {
        # "User modified the Auto Selection. Write to NT variable so robot knows."
        n232 = event-data() -> ("NewVal"=w377:string)  [unwired: 1 in]
        n233 = call <vilib>:"NT Write String.vi"("String"=w377, "Name"="Auto Selector") -> ()  [unwired: 9 in, 1 out]
      }
      event "Command Selection": Value Change {
        # "Get the params and show in table"
        n234 = event-data() -> ("NewVal"=w383:i32)  [unwired: 1 in]
        n235 = property on="Command Selection" class="MCListbox (strict)"() -> ("ItemNames"=w381:string[][])  [unwired: 2 in, 2 out]
        n236 = call <vilib>:"WPI_DashboardUpdate Command Params.vi"("NewVal"=w383, "Commands"=w381, "Param Tbl"=w382) -> ()  [unwired: 8 in, 1 out]
      }
      event "Execute Command": Value Change {
        # "Started one, Unique ID holds\nresponse"
        n237 = event-data() -> ()  [unwired: 1 in, 1 out]
        n238 = property on="Command Selection" class="MCListbox (strict)"() -> ("ItemNames"=w394:string[][])  [unwired: 2 in, 2 out]
        n239 = Index Array(array=w394, index (row)="Command Selection", index (col)=0) -> (element=w392:string)
        n240 = call <vilib>:"Invoke Commands.vi"("Command Params"="Command Params", "Function Name"=w392) -> ("Params"=w388:u8, "Started"=w387:bool)  [unwired: 7 in, 1 out]
        n241 = Array Subset(array="Command Params", length (row)=w388) -> (w389:string[][])  [unwired: 3 in]
        n242 = Select(t="Executing" ("Cmd Status"), s=w387, f="" ("Cmd Status")) -> (s? t:f=→"Cmd Status":string)
      }
      event "Command Selection": Double Click {
        n243 = event-data() -> ("Row"=w402:i32)  [unwired: 1 in]
        n244 = property on="Command Selection" class="MCListbox (strict)"() -> ("ItemNames"=w405:string[][])  [unwired: 2 in, 2 out]
        n245 = local read "Command Params"() -> (w401:string[][])
        n246 = Index Array(array=w405, index (row)=w402, index (col)=0) -> (element=w403:string)
        n247 = call <vilib>:"Invoke Commands.vi"("Command Params"=w401, "Function Name"=w403) -> ("Params"=w400:u8, "Started"=w395:bool)  [unwired: 7 in, 1 out]
        n248 = Array Subset(array=w401, length (row)=w400) -> (w399:string[][])  [unwired: 3 in]
        n249 = Select(t="Executing" ("Cmd Status"), s=w395, f="" ("Cmd Status")) -> (s? t:f=w396:string)
        n250 = local write "Cmd Status"(w396) -> ()
      }
      event "CheckList": Double Click {
        # "Shift clears all"
        # "Update symbols on the listbox"
        n251 = event-data() -> ("PlatMods.Shift"=w407:bool, "Row"=w409:i32)  [unwired: 1 in]
        n252 = case shown="True" w407 {
          tunnel: w409 -> [w413 _]
          tunnel: 1 -> [w412 _]
          frame False {
            n253 = property on="CheckList" class="LstBox (strict)"() -> ("Item Symbols"=w411:i32[])  [unwired: 2 in, 2 out]
            n254 = Replace Array Subset(array=w411, new element=w412, index=w413) -> (w410:i32[])
            n255 = property on="CheckList" class="LstBox (strict)"("Item Symbols"=w410) -> ()  [unwired: 2 in, 2 out]
          }
          frame True {
            w414 = 0 ("Top Row")
            n256 = property on="CheckList" class="LstBox (strict)"() -> ("Number of Rows"=w416:u32)  [unwired: 2 in, 2 out]
            n257 = Initialize Array(0, w416) -> (w415:i32[])
            n258 = property on="CheckList" class="LstBox (strict)"("Top Row"=w414, "Value"=w414, "Item Symbols"=w415) -> ()  [unwired: 2 in, 2 out]
          }
        }
      }
      event "CheckList": Key Down {
        # "Update symbols on the listbox\nLeft and right keys check and uncheck"
        n259 = event-data() -> ("VKey"=w420:T22)  [unwired: 1 in]
        n260 = case shown="\"Left\", \"Right\"" w420 {
          selector: w420 -> [w425 _]
          tunnel: eventvkey."Left" ("VKey") -> [w423 _]
          frame "Left", "Right" {
            n261 = Equal?(x=w423, y=w425) -> (x = y?=w424:bool)
            n262 = Select(t=0, s=w424, f=1) -> (s? t:f=w426:i32)
            n263 = property on="CheckList" class="LstBox (strict)"() -> ("Item Symbols"=w429:i32[])  [unwired: 2 in, 2 out]
            n264 = Replace Array Subset(array=w429, new element=w426, index="CheckList") -> (w428:i32[])
            n265 = property on="CheckList" class="LstBox (strict)"("Item Symbols"=w428) -> ()  [unwired: 2 in, 2 out]
          }
          frame Default {
          }
        }
      }
      event "Motor.Enable": Value Change {
        # "When the test mode otor enable helper is set, update that\ntree row item's value"
        n266 = event-data() -> ("NewVal"=w435:bool)  [unwired: 1 in]
        n267 = Unbundle("Motor") -> ("Value"=w434:dbl)  [unwired: 1 out]
        n268 = Select(t=w434, s=w435, f=0.0) -> (s? t:f=w432:dbl)
        n269 = call <vilib>:"NT Write Number.vi"("Numeric"=w432, "Name"=w431) -> ()  [unwired: 9 in, 1 out]
      }
      event "Test Slider": Value Change {
        # "When the test mode slider helper is set, update that\ntree row item's value"
        n270 = event-data() -> ("NewVal"=w438:dbl)  [unwired: 1 in]
        n271 = call <vilib>:"NT Write Number.vi"("Numeric"=w438, "Name"=w439) -> ()  [unwired: 9 in, 1 out]
      }
      event "On/Off": Value Change {
        # "When the test mode on/off helper value is set, update that\ntree row item's value"
        n272 = event-data() -> ("NewVal"=w443:bool)  [unwired: 1 in]
        n273 = Boolean To (0,1)(Boolean=w443) -> (0, 1=w442:i16)
        n274 = call <vilib>:"NT Write Number.vi"("Numeric"=w442, "Name"=w441) -> ()  [unwired: 9 in, 1 out]
      }
      event "Rev/Fwd": Value Change {
        # "When the test mode helper value for relays is set, update that\ntree row item's value"
        n275 = event-data() -> ("NewVal.Forward"=w451:bool, "NewVal.Reverse"=w450:bool)  [unwired: 1 in]
        n276 = Boolean To (0,1)(Boolean=w451) -> (0, 1=w447:i16)
        n277 = Boolean To (0,1)(Boolean=w450) -> (0, 1=w449:i16)
        n278 = Negate(x=w449) -> (-x=w448:i16)
        n279 = Add(x=w447, y=w448) -> (x+y=w446:i16)
        n280 = call <vilib>:"NT Write Number.vi"("Numeric"=w446, "Name"=w445) -> ()  [unwired: 9 in, 1 out]
      }
      event "Test Ring": Value Change {
        # "When a test mode helper value is selected from the ring,\nset the tree item's variable to the string value"
        n281 = event-data() -> ("NewVal"=w455:u16)  [unwired: 1 in]
        n282 = property on="Test Ring" class="Ring (strict)"() -> ("Strings []"=w456:string[])  [unwired: 2 in, 2 out]
        n283 = Index Array(array=w456, index=w455) -> (element=w454:string)
        n284 = call <vilib>:"NT Write String.vi"("String"=w454, "Name"=w453) -> ()  [unwired: 9 in, 1 out]
      }
      event "Rec Mode": Value Change {
        # "Update globals for recording mode and path to read log from.\nClear when logging and let NetworkTables set path for vision to\nuse."
        n285 = event-data() -> ("NewVal"=w467:enum32{"Stop", "Record", "Playback"})  [unwired: 1 in]
        n286 = global write "WPI_DashboardLogging Global.vi" "Logging Filename"(path "") -> ()
        n287 = global write "WPI_DashboardLogging Global.vi" "Recording"(w467) -> ()
        n288 = case shown="\"Playback\"" w467 {
          tunnel: w466 -> [_ w469 w478]
          tunnel: [_ _ w477] -> w464
          tunnel: [_ _ w476] -> _
          tunnel: w462 -> [_ _ w474]
          tunnel: cluster{i32, i32} {-250, 170} -> [_ _ w473]
          tunnel: [_ _ T23 {"Image Size"=TRUE, "Image Type"=TRUE, "Pixel Value"=TRUE, "ROI Information"=TRUE, "Zoom Factor"=FALSE} ("Image Information Shown:All Elements")] -> w457
          tunnel: [_ _ TRUE ("Zoom Factor")] -> w458
          tunnel: w460 -> [_ _ w470]
          frame Default {
          }
          frame "Stop", "Record" {
            # "Place Window too"
            n289 = invoke class="VI" method="FP.Close"(reference=w469) -> (reference out=w468:refnum<vi>)  [unwired: 2 in, 2 out]
            n290 = invoke class="VI" method="Abort VI"(reference=w468) -> ()  [unwired: 2 in, 3 out]
          }
          frame "Playback" {
            n291 = call "Open Playback Panel.vi"("Offset"=w473, "DB VI Ref"=w474, "Playback in"=w478) -> ("Playback out"=w475:refnum<vi>)  [unwired: 8 in]
            n292 = register-events(w475, w470) -> (reference out=w477:refnum<event-registration>, error out=w476:errorcluster)  [unwired: 2 in]
          }
        }
        n293 = property on="Camera Image Right" class="ImageControl"("Image Information Shown"=w457, "Image Information Visible"=w458) -> ()  [unwired: 2 in, 2 out]
        n294 = property on="Camera Image" class="ImageControl"("Image Information Shown"=w457, "Image Information Visible"=w458) -> ()  [unwired: 2 in, 2 out]
        n295 = call <vilib>:"WPI_DashboardNT Log FieldName Cache.vi"("Operation"=enum16{"Lookup/Add", "Index", "Clear"}."Clear") -> ()  [unwired: 8 in, 3 out]
      }
      event Panel Close {
        w480 = enum32{"Stop", "Record", "Playback"}."Stop" ("Rec Mode")
        # "Playback window has been closed, abort"
        n296 = event-data() -> ()  [unwired: 1 in, 4 out]
        n297 = local write "Rec Mode"(w480) -> ()
        n298 = global write "WPI_DashboardLogging Global.vi" "Recording"(w480) -> ()
      }
      event Panel Close {
        # "Abort playback window and ourself"
        n299 = event-data() -> ()  [unwired: 1 in, 4 out]
        n300 = invoke class="VI" method="FP.Close"(reference=w484) -> (reference out=w483:refnum<vi>)  [unwired: 2 in, 2 out]
        n301 = invoke class="VI" method="Abort VI"(reference=w483) -> (error out=w482:errorcluster)  [unwired: 2 in, 2 out]
        n302 = invoke class="VI" method="Abort VI"(error in=w482) -> ()  [unwired: 2 in, 3 out]
      }
      event User Event {
        n303 = event-data() -> ("IDs"=w491:cluster{"RPC field ID":u16, "Unique ID":u16}, "String"=w490:string)  [unwired: 1 in]
        n304 = Bundle("IDs"=w491, "String"=w490) -> (w489:T10)  [unwired: 1 in]
        n305 = call <vilib>:"Retrieve RPC Response.vi"("RPC Response"=w489) -> ("Output"=w487:string[][])  [unwired: 10 in]
        n306 = Build Array (concatenate)(w485, w487) -> (w486:string[][])
        n307 = local write "Command Params"(w486) -> ()
        n308 = local write "Cmd Status"("" ("Cmd Status")) -> ()
      }
      event "Tree": Double Click {
        n309 = event-data() -> ("PlatMods"=w497:T26, "Tag"=w494:string)  [unwired: 1 in]
        n310 = Unbundle(w497) -> ("Shift"=w496:bool)  [unwired: 4 out]
        n311 = String Subset(string=w494, length (rest)=1 ("length (rest)")) -> (substring=w493:string)  [unwired: 1 in]
        n312 = Not(x=w496) -> (.not. x?=w495:bool)
        n313 = case shown="\"/\"" w493 {
          tunnel: w494 -> [_ w500]
          tunnel: w495 -> [_ w499]
          frame Default {
          }
          frame "/" {
            n314 = call <vilib>:"NT Update Persistence.vi"("Persistence"=w499, "Name"=w500) -> ()  [unwired: 9 in, 1 out]
          }
        }
      }
    }
  }
  n315 = Write to Text File(file (use dialog)=w23, text=w20) -> (refnum out=w22:refnum<file>, error out=w12:errorcluster)  [unwired: 2 in, 1 out]
  n316 = Write to Text File(file (use dialog)=w17, text=w15) -> (refnum out=w16:refnum<file>, error out=w11:errorcluster)  [unwired: 2 in, 1 out]
  n317 = while {
    tunnel: w87 -> [w502]
    i -> [w505]
    stop <- FALSE stop-if-true
    n318 = Wait (ms)(milliseconds to wait=u32 100) -> ()  [unwired: 1 out]
    n319 = case shown="\"Playback\"" "Rec Mode" {
      tunnel: w505 -> [_ _ w520]
      tunnel: [u32 2829099 ("Base Color") u32 11141120 ("Target Color") w509] -> w501
      frame "Stop", Default {
        # "Reset the color, extra updates don't cost much"
      }
      frame "Record" {
      }
      frame "Playback" {
        # "Playback"
        n320 = Quotient & Remainder(x=w520, y=u32 50 ("milliseconds to wait")) -> (x-y*floor(x/y)=w516:u32)  [unwired: 1 out]
        n321 = Divide(x=w516, y=u32 50 ("milliseconds to wait")) -> (x/y=w513:dbl)
        n322 = Multiply(x=6.283185307179586, y=w513) -> (x*y=w518:dbl)
        n323 = Sine(x=w518) -> (sin(x)=w517:dbl)
        n324 = Absolute Value(x=w517) -> (abs(x)=w510:dbl)
        n325 = call "Interpolate RGB Color.vi"("Proportion"=w510, "Target Color"=u32 30976, "Base Color"=u32 2829099) -> ("Result Color"=w509:u32)  [unwired: 8 in]
      }
    }
    n326 = property class="Pane"(reference=w502, "PaneColor"=w501) -> ()  [unwired: 1 in, 2 out]
  }
  n327 = Close File(refnum=w22, error in=w12) -> ()  [unwired: 2 out]
  n328 = Close File(refnum=w16, error in=w11) -> ()  [unwired: 2 out]
  n329 = call-poly <vilib>:"NT Read Value.vi"("Name"="conveyorSensor03") -> ("Boolean"=→"Conveyor Sensor 3":bool)  [unwired: 9 in, 1 out]
  n330 = call-poly <vilib>:"NT Read Value.vi"("Name"="conveyorSensor01") -> ("Boolean"=→"Conveyor Sensor 1":bool)  [unwired: 9 in, 1 out]
  n331 = call-poly <vilib>:"NT Read Value.vi"("Name"="conveyorSensor04") -> ("Boolean"=→"Conveyor Sensor 4":bool)  [unwired: 9 in, 1 out]
  n332 = call-poly <vilib>:"NT Read Value.vi"("Name"="conveyorSensor02") -> ("Boolean"=→"Conveyor Sensor 2":bool)  [unwired: 9 in, 1 out]
  n333 = local write "Dashboard Tab"(T2."Drive" ("Dashboard Tab")) -> ()
  n334 = Read from Text File() -> (refnum out=w9:refnum<file>, error out=w10:errorcluster)  [unwired: 4 in, 2 out]
  n335 = Close File(refnum=w9, error in=w10) -> ()  [unwired: 2 out]
  n336 = property on="On/Off" class="Bool (strict)"("Visible"=w60) -> ()  [unwired: 2 in, 2 out]
  n337 = property on="Motor" class="Clust (strict)"("Visible"=w60) -> ()  [unwired: 2 in, 2 out]
  n338 = property on="Progress" class="Clust (strict)"("Visible"=w60) -> ()  [unwired: 2 in, 2 out]
  n339 = property on="Test Ring" class="Ring (strict)"("Visible"=w60) -> ()  [unwired: 2 in, 2 out]
  n340 = property on="Rev/Fwd" class="Clust (strict)"("Visible"=w60) -> ()  [unwired: 2 in, 2 out]
  n341 = while {
    tunnel: u16 1741 ("timeout ms (25000)") -> [w522]
    stop <- FALSE stop-if-true
    n342 = TCP Create Listener(10:w522) -> (0:w521:errorcluster, 3:w523:refnum<k5>)  [unwired: 4 in, 1 out]
    n343 = case shown="No Error" w521 {
      selector: w521 -> [w525 _]
      tunnel: w523 -> [w526 _]
      frame No Error {
        n344 = while {
          tunnel: w526 -> [w529]
          tunnel: w525 -> [w528]
          stop <- FALSE stop-if-true
          n345 = TCP Wait On Listener(8:w528, 11:w529) -> (0:w530:errorcluster, 4:w531:refnum<k5>)  [unwired: 2 in, 3 out]
          n346 = local write "TCP"(w531) -> ()
          n347 = case shown="No Error" w530 {
            frame No Error {
            }
            frame Error {
              n348 = Wait (ms)(milliseconds to wait=u32 1000) -> ()  [unwired: 1 out]
            }
          }
        }
      }
      frame Error {
        n349 = Wait (ms)(milliseconds to wait=u32 1000) -> ()  [unwired: 1 out]
      }
    }
  }
  n350 = local write "Command Selection"(u16 0 ("milliseconds to wait")) -> ()
  n351 = local write "Command Params"(string[][] [] ("Command Params")) -> ()
  n352 = global write "WPI_DashboardLogging Global.vi" "Recording"(w81) -> ()
  n353 = local write "Rec Mode"(w81) -> ()
  n354 = call <vilib>:"NT Write String.vi"("String"="Select Auto", "Name"="Auto Selector") -> ()  [unwired: 9 in, 1 out]
